vi "Write State_.vi"(10 "State:":T1, 11 "Logger in":refnum<class "Log.lvclass">) -> (3 "Logger out":refnum<class "Log.lvclass">)   [LabVIEW 2013]
uses:
  Log.lvclass
  Typedefs/StateSelector.ctl
  Typedefs/M2AADTTypedefs.lvlib
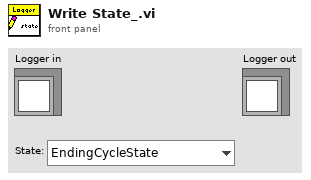
[diagram p1: front panel]
types:
  T1 = typedef "M2AADTTypedefs.lvlib/StateSelector.ctl" = enum16{"EndingCycleState", "FaultState", "InteractiveMotionState", "MovingToNewForceState", "OffState", "PausingState", "StandbyState", "StoppedState"}
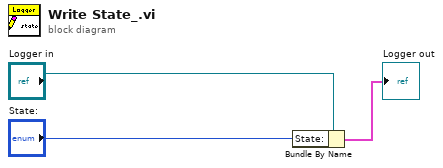
[diagram p0: block diagram]
diagram:
  n1 = Bundle By Name(cluster="Logger in", "State:"="State:") -> (→"Logger out":cluster{})
